vi "Write distance_deg.vi"(8 "error in (no error)":errorcluster, 10 "distance_deg":dbl[unit], 11 "SunMoonStatus in":refnum<class "SunMoonStatus.lvclass">) -> (0 "error out":errorcluster, 3 "SunMoonStatus out":refnum<class "SunMoonStatus.lvclass">)   [LabVIEW 2014, in "TCSDataDefinitions.lvlib" / "TCSPublicStatus.lvlib" / "Limits.lvlib" / "SunMoonStatus.lvclass"]
uses:
  SunMoonStatus.lvclass
  SunMoonStatus.lvclass/SunMoonStatus.ctl
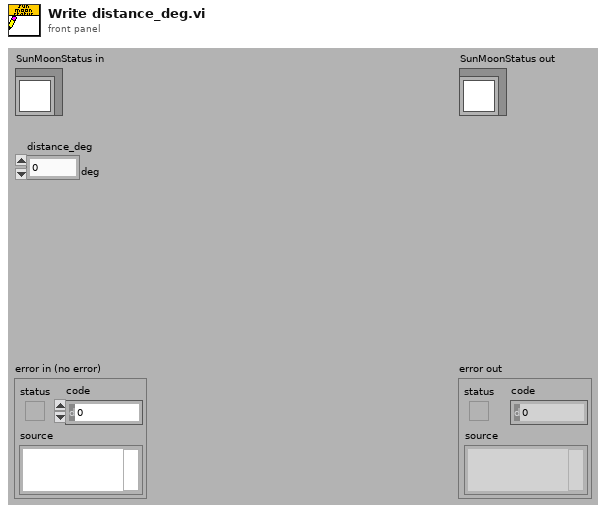
[diagram p1: front panel]
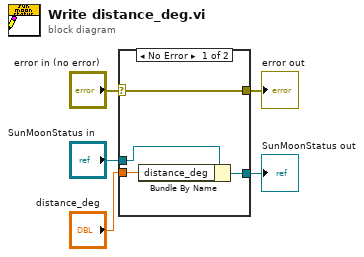
[diagram p0: block diagram]
diagram:
  n1 = case shown="No Error" "error in (no error)" {
    selector: "error in (no error)" -> [w9 w10]
    tunnel: [w9 w10] -> w4
    tunnel: [w7 w11] -> w2
    tunnel: "SunMoonStatus in" -> [w8 w11]
    tunnel: "distance_deg" -> [w6 _]
    frame No Error {
      n2 = Bundle By Name(cluster=w8, "distance_deg"=w6) -> (w7:refnum<class "SunMoonStatus.lvclass">)
    }
    frame Error {
    }
  }
  "error out" <- w4
  "SunMoonStatus out" <- w2
